vi "Write STEP N°.vi"(8 "error in (no error)":errorcluster, 10 "STEP N°":u32, 11 "STEP in":refnum<class "STEP.lvclass">) -> (0 "error out":errorcluster, 3 "STEP out":refnum<class "STEP.lvclass">)   [LabVIEW 2014, in "SeqLoop.lvlib" / "STEP Classes.lvlib" / "STEP.lvclass"]
uses:
  STEP.lvclass
  STEP.lvclass/STEP.ctl
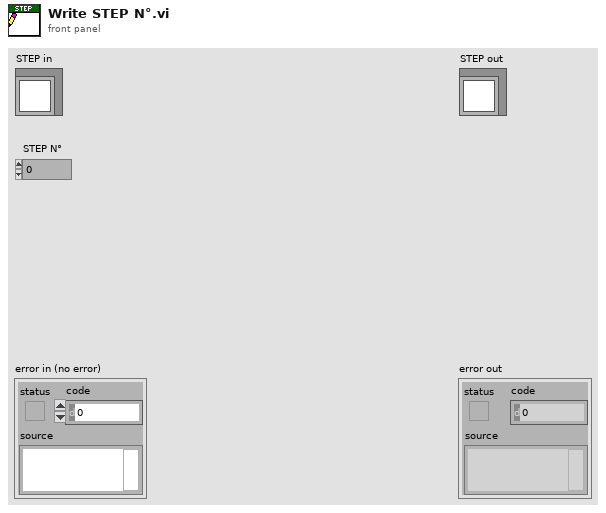
[diagram p1: front panel]
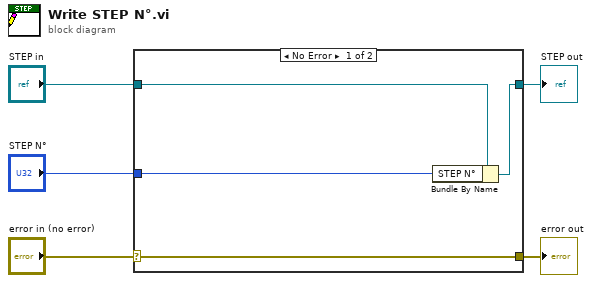
[diagram p0: block diagram]
diagram:
  n1 = case shown="No Error" "error in (no error)" {
    selector: "error in (no error)" -> [w9 w10]
    tunnel: [w9 w10] -> w4
    tunnel: [w7 w11] -> w2
    tunnel: "STEP in" -> [w8 w11]
    tunnel: "STEP N°" -> [w6 _]
    frame No Error {
      n2 = Bundle By Name(cluster=w8, "STEP N°"=w6) -> (w7:refnum<class "STEP.lvclass">)
    }
    frame Error {
    }
  }
  "error out" <- w4
  "STEP out" <- w2
